vi "MODEL SELECTION.vi"() -> ()   [LabVIEW 2017]
uses:
  <vilib>/addons/database/Connection.llb/DB Tools Open Connec (String).vi
  Global/Global 1.vi
  <vilib>/addons/database/NI_Database_API.lvlib
panel:
  out "error out 2":errorcluster
  in  "RECIPE SELECT":string(combo)
  in  "error in (no error)":errorcluster
  in  "Cancel Button":bool
  in  "Save Button":bool
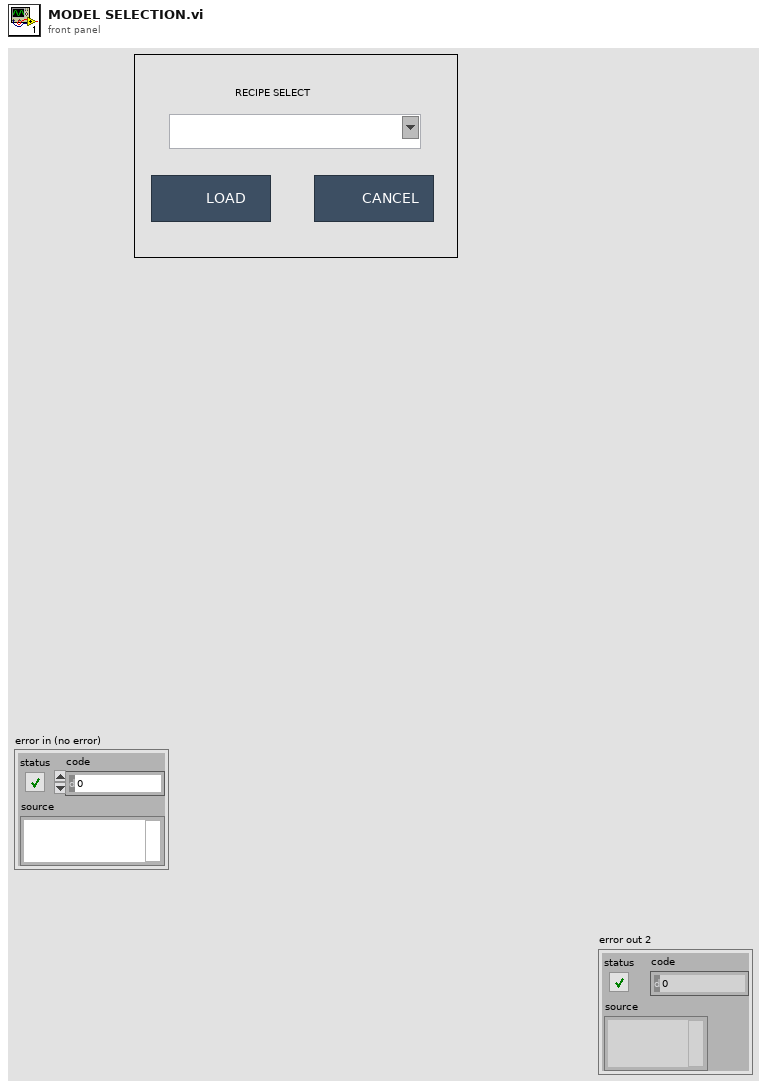
[diagram p1: front panel]
types:
  T1 = typedef "NI_Database_API.lvlib/Conn ObjectReference.ctl" = refnum<k1>
  T2 = enum32{"invalid app kind", "Development System", "Run Time System", "Student Edition", "Embedded LabVIEW", "Evaluation", "Custom"}
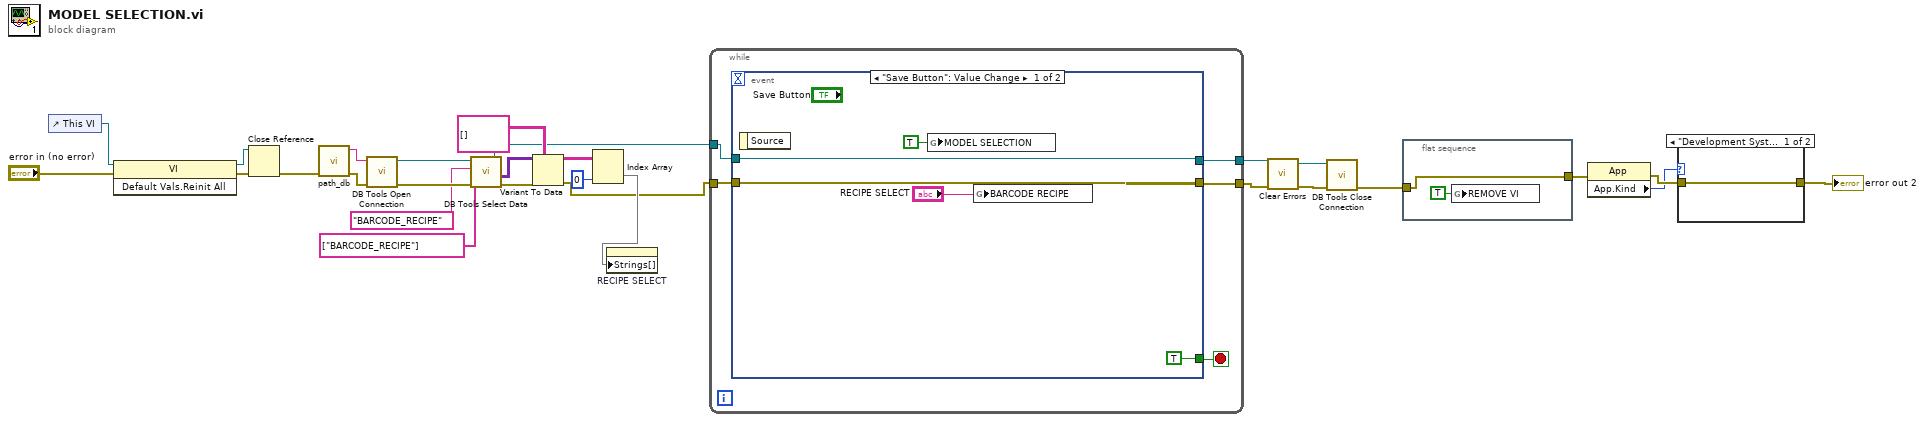
[diagram p0: block diagram]
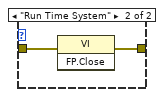
[diagram p2: hidden frame]
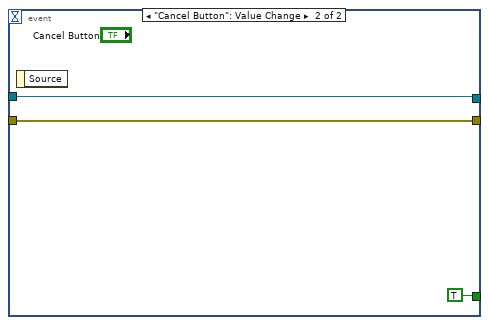
[diagram p3: hidden frame]
diagram:
  n1 = control-ref of="This VI"() -> (w15:refnum<vi>)
  n2 = invoke class="VI" method="Default Vals.Reinit All"(reference=w15, error in="error in (no error)") -> (reference out=w13:refnum<vi>, error out=w12:errorcluster)  [unwired: 1 in, 1 out]
  n3 = Close Reference(reference=w13, error in (no error)=w12) -> (error out=w10:errorcluster)
  n4 = call "path_db.vi"("error in"=w10) -> ("error out"=w11:errorcluster, "resulting string"=w9:string)  [unwired: 9 in]
  n5 = call-poly <vilib>:"DB Tools Open Connection.vi"("error in (no error)"=w11, "connection information"=w9) -> ("error out"=w25:errorcluster, "connection reference"=w24:T1)  [unwired: 6 in]
  n6 = call <vilib>:"DB Tools Select Data.vi"("error in (no error)"=w25, "columns"=string[] ["BARCODE_RECIPE"], "table"="BARCODE_RECIPE", "connection reference"=w24) -> ("error out"=w27:errorcluster, "data"=w26:variant[][], "connection reference out"=w19:T1)  [unwired: 2 in]
  n7 = Variant To Data(error in=w27, type=string[][] [], Variant=w26) -> (data=w21:string[][], error out=w6:errorcluster)
  n8 = Index Array(array=w21, index (col)=0 ("disabled index (col)")) -> (element=w8:string[])  [unwired: 1 in]
  n9 = property on="RECIPE SELECT" class="CmbBox"("Strings[]"=w8) -> ()  [unwired: 2 in, 2 out]
  n10 = while {
    tunnel: w6 -> [w30]
    tunnel: [w31] -> w16
    tunnel: w19 -> [w29]
    tunnel: [w28] -> w18
    stop <- w32 stop-if-true
    n11 = event shown="[0] \"Save Button\": Value Change" {
      selector: _ -> [_ _]
      dyn-events: _ -> [_ _]
      timeout: _ -> [_ _]
      tunnel: [TRUE TRUE] -> w32
      tunnel: [w36 w39] -> w31
      tunnel: w30 -> [w36 w39]
      tunnel: [w35 w38] -> w28
      tunnel: w29 -> [w35 w38]
      event "Save Button": Value Change {
        n12 = event-data() -> ()  [unwired: 1 in, 1 out]
        n13 = global write "Global 1.vi" "MODEL SELECTION"(TRUE ("MODEL SELECTION")) -> ()
        n14 = global write "Global 1.vi" "BARCODE RECIPE"("RECIPE SELECT") -> ()
      }
      event "Cancel Button": Value Change {
        n15 = event-data() -> ()  [unwired: 1 in, 1 out]
      }
    }
  }
  n16 = call <vilib>:"Clear Errors.vi"("error in (no error)"=w16) -> ("error out"=w17:errorcluster)  [unwired: 5 in, 1 out]
  n17 = call <vilib>:"DB Tools Close Connection.vi"("error in (no error)"=w17, "connection reference"=w18) -> ("error out"=w1:errorcluster)  [unwired: 5 in]
  n18 = flat-sequence {
    tunnel: [w41] -> w2
    tunnel: w1 -> [w41]
    frame #0 {
      n19 = global write "Global 1.vi" "REMOVE VI"(TRUE ("remove_VI")) -> ()
    }
  }
  n20 = property class="App"(error in=w2) -> (error out=w4:errorcluster, "App.Kind"=w3:T2)  [unwired: 1 in, 1 out]
  n21 = case shown="\"Development System\", Default" w3 {
    tunnel: [w43 w45] -> w5
    tunnel: w4 -> [w43 w44]
    frame "Development System", Default {
    }
    frame "Run Time System" {
      n22 = invoke class="VI" method="FP.Close"(error in=w44) -> (error out=w45:errorcluster)  [unwired: 2 in, 2 out]
    }
  }
  "error out 2" <- w5
